vi "checkifsmallerthan-400subVI.vi"(10 "port_number in":string, 11 "function return":i32) -> ()   [LabVIEW 2012]
uses:
  <userlib>/SPECcon/SPECcon.lvlib
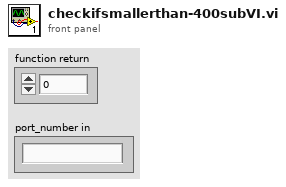
[diagram p1: front panel]
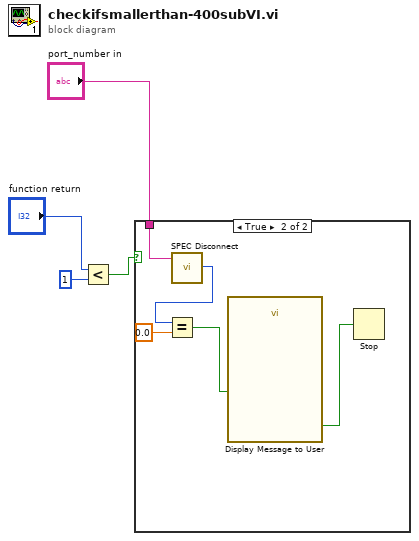
[diagram p0: block diagram]
diagram:
  n1 = Less?(x="function return", y=1) -> (x < y?=w2:bool)
  n2 = case shown="True" w2 {
    tunnel: "port_number in" -> [_ w6]
    frame False {
    }
    frame True {
      n3 = call <userlib>:"SPEC Disconnect.vi"("port_number"=w6) -> ("function return"=w5:i32)  [unwired: 9 in, 1 out]
      n4 = Equal?(x=w5, y=0.0) -> (x = y?=w9:bool)
      n5 = call "Display Message to User"("Enable"=w9) -> ("OK"=w7:bool)  [unwired: 9 in, 1 out]
      n6 = Stop(stop? (T)=w7) -> ()
    }
  }
